vi "Initialize Hardware References.vi"(8 "error in (no error)":errorcluster, 11 "DAQmx Container In":T1) -> (0 "error out":errorcluster, 3 "DAQmx Container Out":T1)   [LabVIEW 2024]
doc: "Initialize the hardware references."
uses:
  support/Control/DAQmx Container.ctl
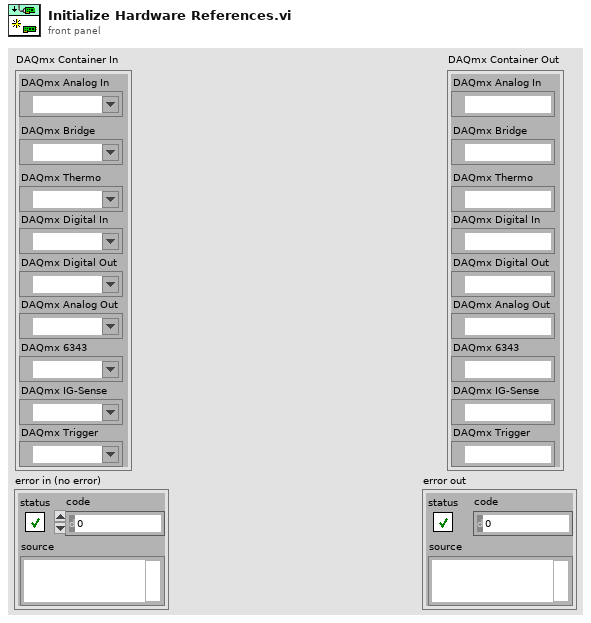
[diagram p1: front panel]
types:
  T1 = typedef "DAQmx Container.ctl" = cluster{"DAQmx Analog In":refnum<k21>, "DAQmx Digital In":refnum<k21>, "DAQmx Digital Out":refnum<k21>, "DAQmx Analog Out":refnum<k21>, "DAQmx 6343":refnum<k21>, "DAQmx IG-Sense":refnum<k21>, "DAQmx Thermo":refnum<k21>, "DAQmx Bridge":refnum<k21>, "DAQmx Trigger":refnum<k21>}
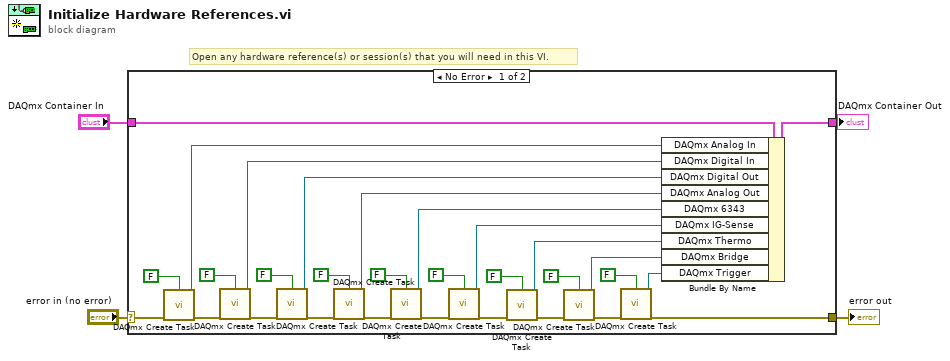
[diagram p0: block diagram]
diagram:
  # "Open any hardware reference(s) or session(s) that you will need in this VI."
  n1 = case shown="No Error" "error in (no error)" {
    selector: "error in (no error)" -> [w31 w35]
    tunnel: [w6 w35] -> w3
    tunnel: "DAQmx Container In" -> [w33 w36]
    tunnel: [w34 w36] -> w1
    frame No Error {
      n2 = call <vilib>:"DAQmx Create Task.vi"("auto cleanup"=FALSE, "error in"=w31) -> ("task out"=w30:refnum<k21>, "error out"=w13:errorcluster)  [unwired: 12 in]
      n3 = call <vilib>:"DAQmx Create Task.vi"("auto cleanup"=FALSE, "error in"=w13) -> ("task out"=w12:refnum<k21>, "error out"=w14:errorcluster)  [unwired: 12 in]
      n4 = call <vilib>:"DAQmx Create Task.vi"("auto cleanup"=FALSE, "error in"=w14) -> ("task out"=w17:refnum<k21>, "error out"=w16:errorcluster)  [unwired: 12 in]
      n5 = call <vilib>:"DAQmx Create Task.vi"("auto cleanup"=FALSE, "error in"=w16) -> ("task out"=w19:refnum<k21>, "error out"=w21:errorcluster)  [unwired: 12 in]
      n6 = call <vilib>:"DAQmx Create Task.vi"("auto cleanup"=FALSE, "error in"=w21) -> ("task out"=w20:refnum<k21>, "error out"=w22:errorcluster)  [unwired: 12 in]
      n7 = call <vilib>:"DAQmx Create Task.vi"("auto cleanup"=FALSE, "error in"=w22) -> ("task out"=w24:refnum<k21>, "error out"=w23:errorcluster)  [unwired: 12 in]
      n8 = call <vilib>:"DAQmx Create Task.vi"("auto cleanup"=FALSE, "error in"=w23) -> ("task out"=w28:refnum<k21>, "error out"=w10:errorcluster)  [unwired: 12 in]
      n9 = call <vilib>:"DAQmx Create Task.vi"("auto cleanup"=FALSE, "error in"=w10) -> ("task out"=w9:refnum<k21>, "error out"=w7:errorcluster)  [unwired: 12 in]
      n10 = call <vilib>:"DAQmx Create Task.vi"("auto cleanup"=FALSE, "error in"=w7) -> ("task out"=w5:refnum<k21>, "error out"=w6:errorcluster)  [unwired: 12 in]
      n11 = Bundle By Name(cluster=w33, "DAQmx Analog In"=w30, "DAQmx Digital In"=w12, "DAQmx Digital Out"=w17, "DAQmx Analog Out"=w19, "DAQmx 6343"=w20, "DAQmx IG-Sense"=w24, "DAQmx Thermo"=w28, "DAQmx Bridge"=w9, "DAQmx Trigger"=w5) -> (w34:T1)
    }
    frame Error {
    }
  }
  "error out" <- w3
  "DAQmx Container Out" <- w1
